vi "configurationFileKeys.vi"() -> (1 "configKeysRT":string[][](array[string])=[["system", "configFileVersionID"], ["messageHandler", "none"], ["FIFO", "none"], ["comms", "errorWriterName"], ["comms", "commandReaderName"], ["comms", "errorBufferSize"], ["comms", "commandBufferSize"], ["comms", "scanivalveIP"], ["comms", "scanPeriod"], ["dataProcessor", "totalChannels"], ["dataProcessor", "dataWriterName"], ["dataProcessor", "NetStreamWriteBufferSize"], ["dataProcessor", "NetStreamBufferLength"]], 2 "write user key?":bool[](array[boolean]), 3 "userConfigKeys":string[][](array[string]))   [LabVIEW 2018]
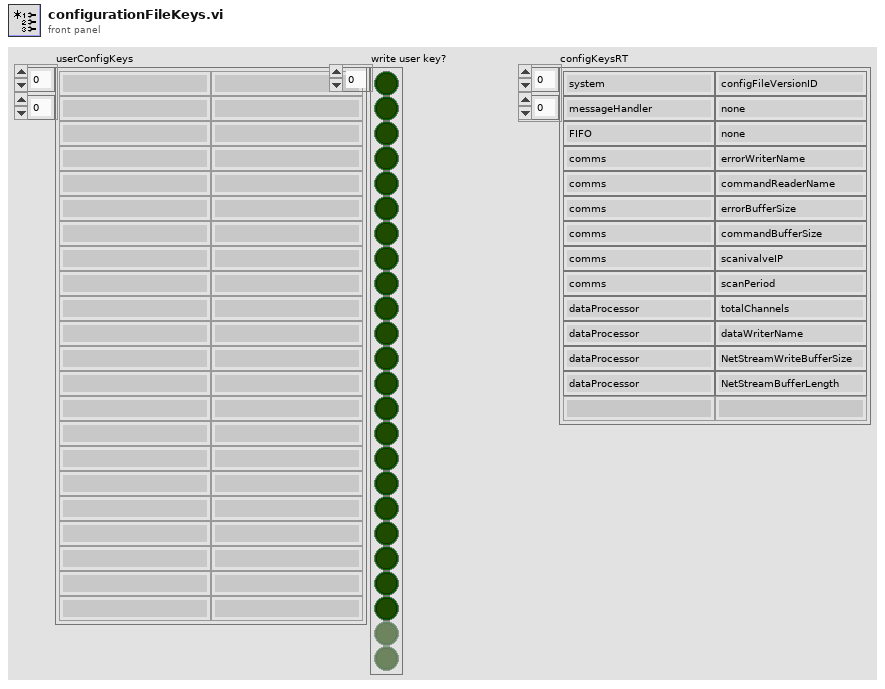
[diagram p1: front panel]
types:
  T1 = cluster{"userConfigKeys":string[], "writeUserKey":bool}[]
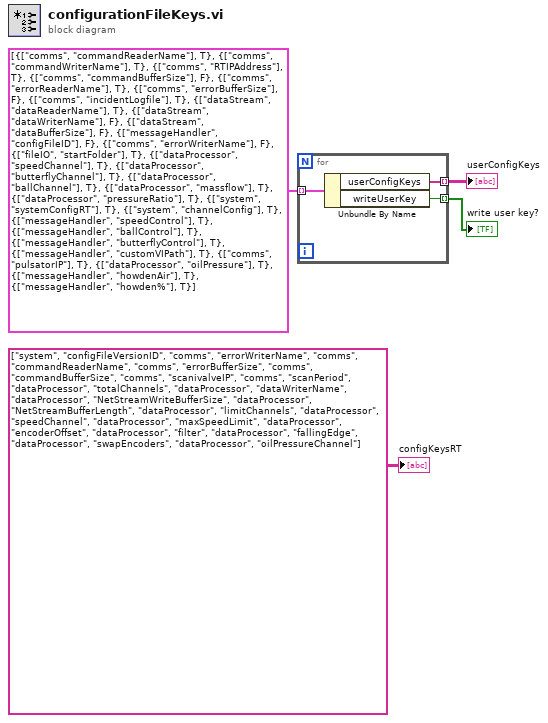
[diagram p0: block diagram]
diagram:
  n1 = for {
    tunnel: T1 [{"userConfigKeys"=["comms", "commandReaderName"], "writeUserKey"=TRUE}, {"userConfigKeys"=["comms", "commandWriterName"], "writeUserKey"=TRUE}, {"userConfigKeys"=["comms", "RTIPAddress"], "writeUserKey"=TRUE}, {"userConfigKeys"=["comms", "commandBufferSize"], "writeUserKey"=FALSE}, {"userConfigKeys"=["comms", "errorReaderName"], "writeUserKey"=TRUE}, {"userConfigKeys"=["comms", "errorBufferSize"], "writeUserKey"=FALSE}, {"userConfigKeys"=["comms", "incidentLogfile"], "writeUserKey"=TRUE}, {"userConfigKeys"=["dataStream", "dataReaderName"], "writeUserKey"=TRUE}, {"userConfigKeys"=["dataStream", "dataWriterName"], "writeUserKey"=FALSE}, {"userConfigKeys"=["dataStream", "dataBufferSize"], "writeUserKey"=FALSE}, {"userConfigKeys"=["messageHandler", "configFileID"], "writeUserKey"=FALSE}, {"userConfigKeys"=["comms", "errorWriterName"], "writeUserKey"=FALSE}, {"userConfigKeys"=["fileIO", "startFolder"], "writeUserKey"=TRUE}, {"userConfigKeys"=["dataProcessor", "speedChannel"], "writeUserKey"=TRUE}, {"userConfigKeys"=["dataProcessor", "butterflyChannel"], "writeUserKey"=TRUE}, {"userConfigKeys"=["dataProcessor", "ballChannel"], "writeUserKey"=TRUE}, {"userConfigKeys"=["dataProcessor", "massflow"], "writeUserKey"=TRUE}, {"userConfigKeys"=["dataProcessor", "pressureRatio"], "writeUserKey"=TRUE}, {"userConfigKeys"=["system", "systemConfigRT"], "writeUserKey"=TRUE}, {"userConfigKeys"=["system", "channelConfig"], "writeUserKey"=TRUE}, {"userConfigKeys"=["messageHandler", "speedControl"], "writeUserKey"=TRUE}, {"userConfigKeys"=["messageHandler", "ballControl"], "writeUserKey"=TRUE}, {"userConfigKeys"=["messageHandler", "butterflyControl"], "writeUserKey"=TRUE}, {"userConfigKeys"=["messageHandler", "customVIPath"], "writeUserKey"=TRUE}, {"userConfigKeys"=["comms", "pulsatorIP"], "writeUserKey"=TRUE}, {"userConfigKeys"=["dataProcessor", "oilPressure"], "writeUserKey"=TRUE}, {"userConfigKeys"=["messageHandler", "howdenAir"], "writeUserKey"=TRUE}, {"userConfigKeys"=["messageHandler", "howden%"], "writeUserKey"=TRUE}] ("Array 2") -> [w7] mode=indexing
    tunnel: [w6] -> w2 mode=indexing
    tunnel: [w5] -> w1 mode=indexing
    n2 = Unbundle By Name(w7) -> ("userConfigKeys"=w6:string[], "writeUserKey"=w5:bool)
  }
  "userConfigKeys" <- w2
  "write user key?" <- w1
  "configKeysRT" <- string[][] [["system", "configFileVersionID"], ["comms", "errorWriterName"], ["comms", "commandReaderName"], ["comms", "errorBufferSize"], ["comms", "commandBufferSize"], ["comms", "scanivalveIP"], ["comms", "scanPeriod"], ["dataProcessor", "totalChannels"], ["dataProcessor", "dataWriterName"], ["dataProcessor", "NetStreamWriteBufferSize"], ["dataProcessor", "NetStreamBufferLength"], ["dataProcessor", "limitChannels"], ["dataProcessor", "speedChannel"], ["dataProcessor", "maxSpeedLimit"], ["dataProcessor", "encoderOffset"], ["dataProcessor", "filter"], ["dataProcessor", "fallingEdge"], ["dataProcessor", "swapEncoders"], ["dataProcessor", "oilPressureChannel"]] ("appended array 2")
